vi "CustomBeep.vi"(0 "Holding time":dbl=101.0, 1 "Threshold to Beep":dbl=100.0) -> ()   [LabVIEW 2015]
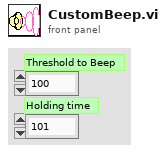
[diagram p1: front panel]
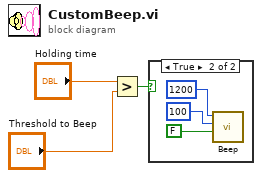
[diagram p0: block diagram]
diagram:
  n1 = Greater?(x="Holding time", y="Threshold to Beep") -> (0:w3:bool)
  n2 = case shown="True" w3 {
    frame False {
    }
    frame True {
      n3 = call <vilib>:"Beep.vi"("use system alert? (T)"=FALSE, "duration (msec)"=u32 100, "frequency (Hz)"=u32 1200) -> ()  [unwired: 9 in]
    }
  }
